vi "PH_Trendviewer_Powermeter.get Powermeters.vi"(0 "i ref in":refnum<vi>, 5 "error in":errorcluster) -> (14 "i ref out":refnum<vi>, 17 "No Powermeter selected?":bool, 19 "error out":errorcluster)   [LabVIEW 2014, in "PH_Trendviewer_Powermeter.lvlib"]
doc: "This VI queries all Image Operator Instances from the data base. Aterwards it indicates in an GUI which of these instances are running tp allow the user to do a selection."
uses:
  PH_Trendviewer_Powermeter.lvlib
  CSCore/CSSystem/CSSystemLib/CSSystemLib.lvlib
  PH_Common/PH_Common.lvlib
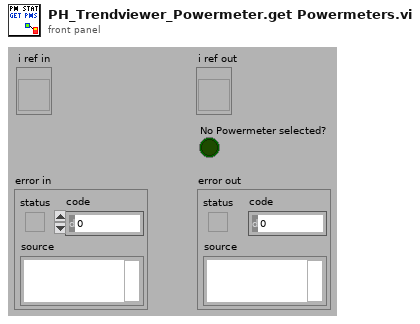
[diagram p1: front panel]
types:
  T1 = typedef "PH_Trendviewer_Powermeter.lvlib/PH_Trendviewer_Powermeter.i attribute.ctl" = cluster{"GUI Refs ":cluster{"Status":refnum<vi>, "Result Graph":refnum<vi>, "Mean Data":refnum<vi>, "Std Dev Data":refnum<vi>, "Dummy Mean":refnum<vi>, "Dummy Std Dev":refnum<vi>, "Export Data":refnum<vi>, "Stat or Trend":refnum<vi>, "Delete":refnum<vi>, "Powermeter":refnum<vi>, "Start":refnum<vi>}, "Powermeter":string, "Stat or Trend":bool, "Start":bool, "Data":cluster{"Time Stamp":timestamp, "Energy [J]":dbl}[], "Datasets strored":i32, "Dataarray Size":i32}
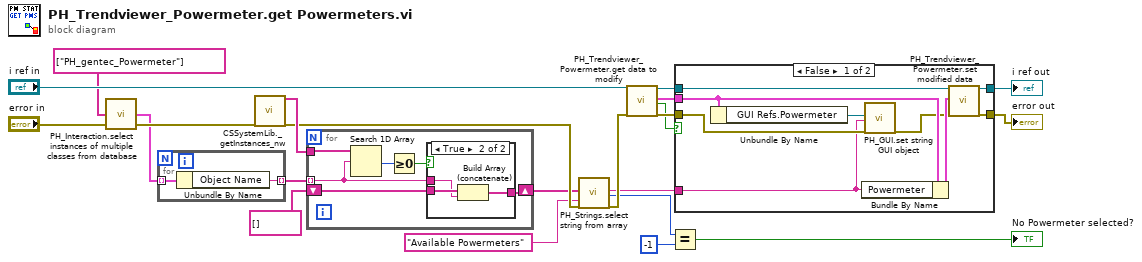
[diagram p0: block diagram]
diagram:
  n1 = call "PH_Interaction.select instances of multiple classes from database.vi"("error in (no error)"="error in", "Classes Input"=string[] ["PH_gentec_Powermeter"]) -> ("error out"=w15:errorcluster, "Query Result"=w13:cluster{"Object Name":string, "Class":string}[])  [unwired: 2 in]
  n2 = for {
    tunnel: w13 -> [w24] mode=indexing
    tunnel: [w23] -> w12 mode=indexing
    n3 = Unbundle By Name(w24) -> ("Object Name"=w23:string)
  }
  n4 = call "CSSystemLib._getInstances_nw.vi"("error in (no error)"=w15) -> ("i list"=w17:string[], "error out"=w8:errorcluster)  [unwired: 17 in]
  n5 = for {
    tunnel: w12 -> [w25] mode=indexing
    shift-right: [w29] -> w5
    shift-left: string[] [] ("Query Result") -> [w30]
    tunnel: w17 -> [w26]
    n6 = Search 1D Array(1D array=w26, element=w25) -> (index of element=w27:i32)  [unwired: 1 in]
    n7 = Greater Or Equal To 0?(x=w27) -> (x >= 0?=w28:bool)
    n8 = case shown="True" w28 {
      tunnel: w30 -> [w31 w34]
      tunnel: [w31 w33] -> w29
      tunnel: w25 -> [_ w32]
      frame False {
      }
      frame True {
        n9 = Build Array (concatenate)(w34, w32) -> (w33:string[])
      }
    }
  }
  n10 = call "PH_Strings.select string from array.vi"("String Array in"=w5, "Caption.Text"="Available Powermeters", "error in (no error)"=w8) -> ("string out"=w4:string, "index"=w3:i32, "error out"=w7:errorcluster)  [unwired: 14 in]
  n11 = call "PH_Trendviewer_Powermeter.get data to modify.vi"("i ref in"="i ref in", "error in (no error)"=w7) -> ("i ref out"=w22:refnum<vi>, "i attribute"=w21:T1, "timed out"=w9:bool, "error out"=w20:errorcluster)  [unwired: 14 in]
  n12 = Equal?(x=w3, y=-1) -> (x = y?=→"No Powermeter selected?":bool)
  n13 = case shown="False" w9 {
    tunnel: w22 -> [w43 w45]
    tunnel: w21 -> [w40 _]
    tunnel: w20 -> [w38 w44]
    tunnel: w4 -> [w35 _]
    tunnel: [w42 w45] -> w11
    tunnel: [w41 w44] -> w10
    frame False {
      n14 = Unbundle By Name(w40) -> ("GUI Refs.Powermeter"=w36:refnum<vi>)
      n15 = Bundle By Name(cluster=w40, "Powermeter"=w35) -> (w39:T1)
      n16 = call "PH_GUI.set string GUI object.vi"("GUI object Ref"=w36, "Text"=w35, "error in"=w38) -> ("error out"=w37:errorcluster)  [unwired: 16 in]
      n17 = call "PH_Trendviewer_Powermeter.set modified data.vi"("i ref in"=w43, "i attribute"=w39, "error in (no error)"=w37) -> ("i ref out"=w42:refnum<vi>, "error out"=w41:errorcluster)  [unwired: 15 in]
    }
    frame True {
    }
  }
  "i ref out" <- w11
  "error out" <- w10
